vi "State_Machine.vi"(8 "error in (no error)":errorcluster caption="entrée d'erreur (pas d'erreur)", 11 "Delay en entrée":refnum<class "P1833_Scan_QRCode.lvclass">) -> (0 "error out":errorcluster caption="sortie d'erreur", 2 "Json_String":string, 3 "Delay en sortie":refnum<class "P1833_Scan_QRCode.lvclass">)   [LabVIEW 2020, in "Library Test.lvlib" / "P1833_Scan_QRCode.lvclass"]
uses:
  P1833_Scan_QRCode.lvclass
  C:/Users/ngarcin/OneDrive - Altyor/Standard TB/Suite TB45/Class/Test/Test (Default)/Test (Default).lvclass
  Popup/Class Popup Operator_Input Batch_AIS/Class Popup Operator_Input_PCRE.lvclass
  Commun VI/TypeDef/Variable Printable.ctl
  Popup/Class Popup (Main)/Class Popup (Main).lvclass
  JSON API/JSON Value/Set from JSON string.vi
  JSON API/JSON Value/JSON Value.lvclass
  JSON API/Variant JSON/Variant JSON.lvlib
  JSON API/Get Polymorphic/JSON GetSet.lvlib
  Commun VI/Library Commun.lvlib
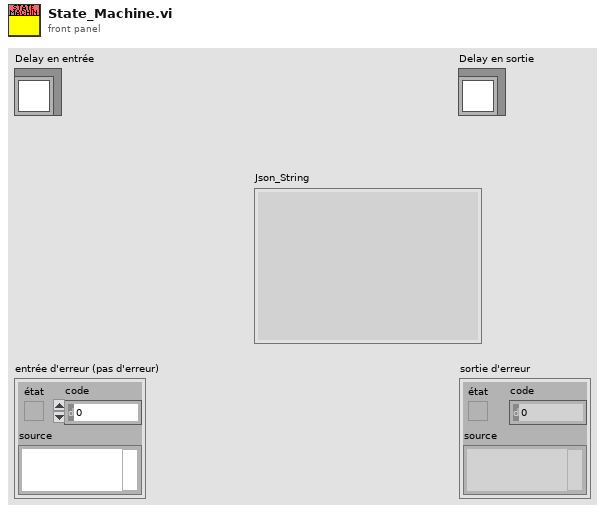
[diagram p1: front panel]
types:
  T1 = typedef "Variable Printable.ctl" = string
  T2 = enum16{"Get Variable", "Get All Variables", "Set Variable", "Delete Variable", "Delete All Variable"}
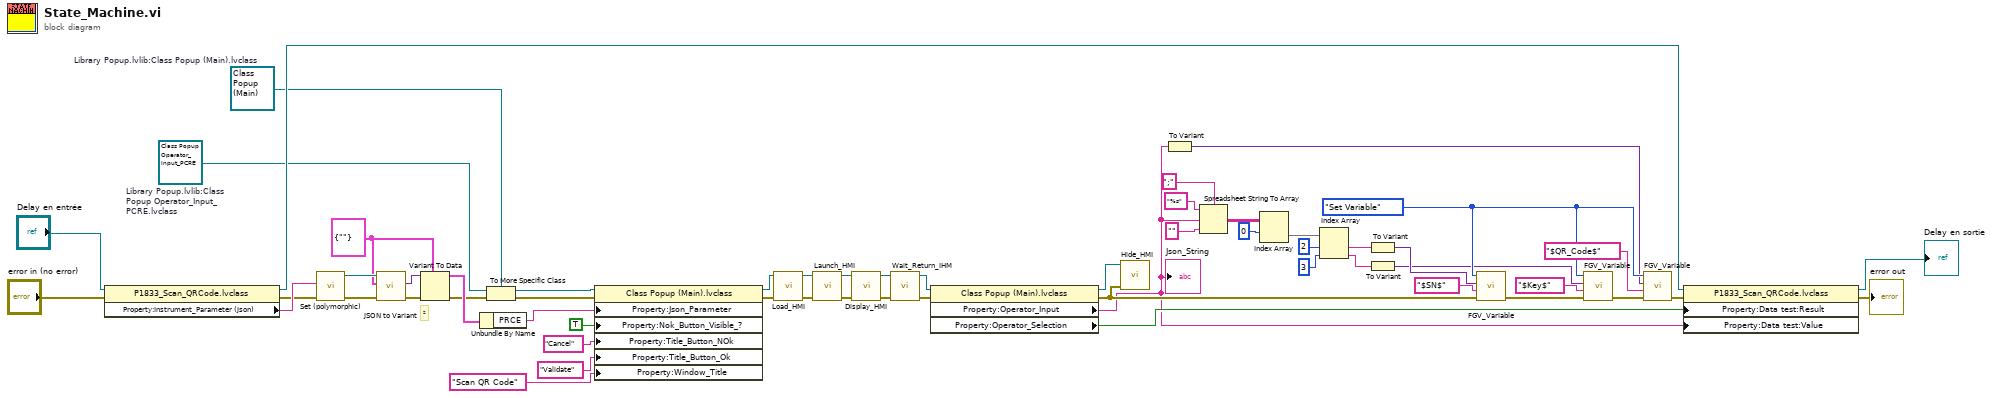
[diagram p0: block diagram]
diagram:
  w26 = refnum<class "Class Popup (Main).lvclass"> refnum  # Library Popup.lvlib:Class Popup (Main).lvclass
  w16 = T2."Set Variable" ("Function")
  w32 = cluster{"PRCE":string} {"PRCE"=""}
  w25 = refnum<class "Class Popup Operator_Input_PCRE.lvclass"> refnum  # Library Popup.lvlib:Class Popup Operator_Input_PCRE.lvclass
  # "²"
  n1 = property class="P1833_Scan_QRCode.lvclass"(reference="Delay en entrée", error in="error in (no error)") -> (reference out=w38:refnum<class "P1833_Scan_QRCode.lvclass">, error out=w54:errorcluster, "Property:Instrument_Parameter (Json)"=w56:string)
  n2 = call-poly "Set (polymorphic).vi"("error in (no error)"=w54, "JSON stream"=w56) -> ("error out"=w34:errorcluster, "JSON Value out"=w36:refnum<class "JSON Value.lvclass">)  [unwired: 7 in, 1 out]
  n3 = call "JSON to Variant.vi"("error in (no error)"=w34, "Variant (Data Type)"=w32, "JSON Value"=w36) -> ("error out"=w35:errorcluster, "Variant out"=w33:variant)  [unwired: 7 in]
  n4 = Variant To Data(error in=w35, type=w32, Variant=w33) -> (data=w31:cluster{"PRCE":string}, error out=w23:errorcluster)
  n5 = Unbundle By Name(w31) -> ("PRCE"=w30:string)
  n6 = To More Specific Class(target class=w26, reference=w25, error in=w23) -> (specific class reference=w24:refnum<class "Class Popup (Main).lvclass">, error out=w22:errorcluster)
  n7 = property class="Class Popup (Main).lvclass"(reference=w24, error in=w22, "Property:Json_Parameter"=w30, "Property:Nok_Button_Visible_?"=TRUE ("Nok_Button_Visible_?"), "Property:Title_Button_NOk"="Cancel" ("Title_Button_NOk"), "Property:Title_Button_Ok"="Validate" ("Title_Button_Ok"), "Property:Window_Title"="Scan QR Code" ("Window_Title")) -> (reference out=w48:refnum<class "Class Popup (Main).lvclass">, error out=w47:errorcluster)
  n8 = call-dynamic "Load_HMI.vi"("error in (no error)"=w47, "Class Popup (Default) en entrée"=w48) -> ("error out"=w53:errorcluster, "Class Popup (Default) en sortie"=w52:refnum<class "Class Popup (Main).lvclass">)  [unwired: 8 in]
  n9 = call-dynamic "Launch_HMI.vi"("error in (no error)"=w53, "Class Popup (Default) en entrée"=w52) -> ("error out"=w51:errorcluster, "Class Popup (Default) en sortie"=w50:refnum<class "Class Popup (Main).lvclass">)  [unwired: 8 in]
  n10 = call-dynamic "Display_HMI.vi"("error in (no error)"=w51, "Class Popup (Default) en entrée"=w50) -> ("error out"=w20:errorcluster, "Class Popup (Default) en sortie"=w49:refnum<class "Class Popup (Main).lvclass">)  [unwired: 8 in]
  n11 = call-dynamic "Wait_Return_IHM.vi"("error in (no error)"=w20, "Class Popup (Default) en entrée"=w49) -> ("error out"=w21:errorcluster, "Class Popup (Default) en sortie"=w43:refnum<class "Class Popup (Main).lvclass">)  [unwired: 8 in]
  n12 = property class="Class Popup (Main).lvclass"(reference=w43, error in=w21) -> (reference out=w42:refnum<class "Class Popup (Main).lvclass">, error out=w19:errorcluster, "Property:Operator_Input"=w2:string, "Property:Operator_Selection"=w37:bool)
  "Json_String" <- w2
  n13 = call-dynamic "Hide_HMI.vi"("error in (no error)"=w19, "Class Popup (Default) en entrée"=w42) -> ()  [unwired: 8 in, 2 out]
  n14 = To Variant(anything=w2) -> (Variant=w1:variant)
  n15 = Spreadsheet String To Array(delimiter (Tab)=";" ("séparateur (Tabulation)"), format string="%s" ("chaîne de format"), spreadsheet string=w2, array type (2D Dbl)="") -> (array=w9:string[][])
  n16 = Index Array(array=w9, index (row)=0 ("indice (ligne)")) -> (element=w8:string[])  [unwired: 1 in]
  n17 = Index Array(array=w8, index #1=2 ("indice"), index #2=3 ("indice")) -> (element #1=w5:string, element #2=w4:string)
  n18 = To Variant(anything=w5) -> (Variant=w17:variant)
  n19 = To Variant(anything=w4) -> (Variant=w3:variant)
  n20 = call "FGV_Variable.vi"("error in (no error)"=w19, "Variable"=T1 "$SN$", "Data In"=w17, "Function"=w16) -> ("error out"=w18:errorcluster)  [unwired: 5 in, 2 out]
  n21 = call "FGV_Variable.vi"("error in (no error)"=w18, "Variable"=T1 "$Key$", "Data In"=w3, "Function"=w16) -> ("error out"=w28:errorcluster)  [unwired: 5 in, 2 out]
  n22 = call "FGV_Variable.vi"("error in (no error)"=w28, "Variable"=T1 "$QR_Code$" ("Variable Printable"), "Data In"=w1, "Function"=w16) -> ("error out"=w14:errorcluster)  [unwired: 5 in, 2 out]
  n23 = property class="P1833_Scan_QRCode.lvclass"(reference=w38, error in=w14, "Property:Data test:Result"=w37, "Property:Data test:Value"=w2) -> (reference out=→"Delay en sortie":refnum<class "P1833_Scan_QRCode.lvclass">, error out=→"error out":errorcluster)
